vi "DUTResultsDialogSequential.vi"(5 "Left Coordinate":i16, 7 "Top Coordinate":i16, 8 "error in (no error)":errorcluster, 9 "MessageTxt":string, 11 "Value":string) -> (0 "error out":errorcluster)   [LabVIEW 2021]
doc: "Display DUT results banner for Pass, Fail, Error or Terminate."
panel:
  out "MssgText":string
  out "Message":string
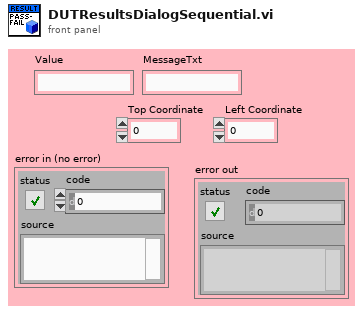
[diagram p1: front panel]
types:
  T1 = typedef "imagedata.ctl" = cluster{"image type":i32, "image depth":i32, "image":u8[], "mask":u8[], "colors":u32[], "Rectangle":cluster{"left":i16, "top":i16, "right":i16, "bottom":i16}}
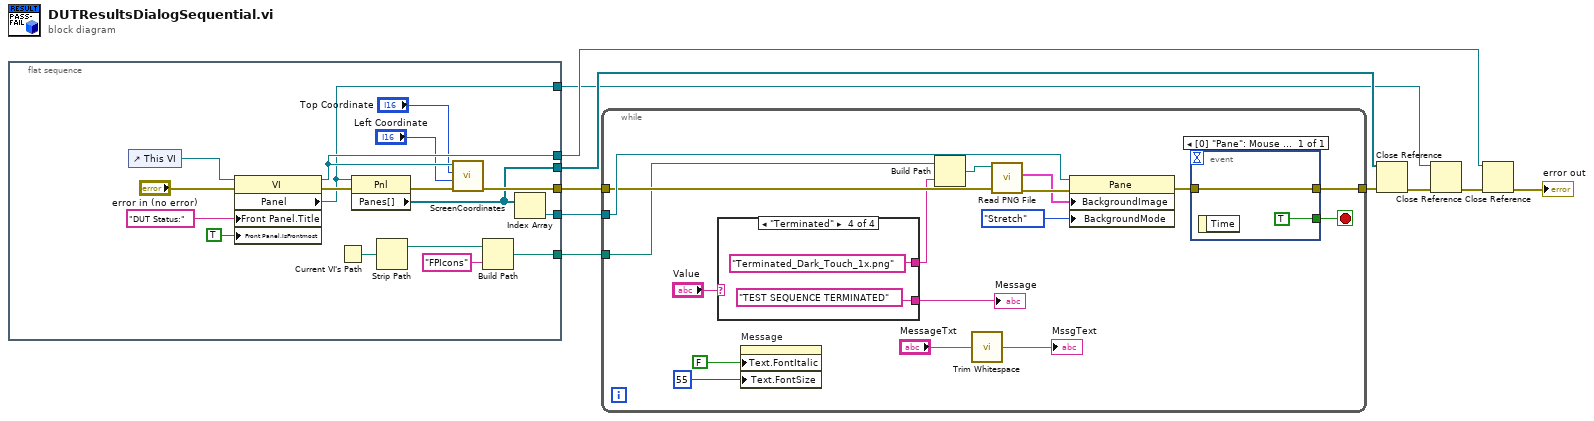
[diagram p0: block diagram]
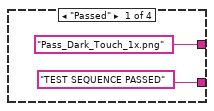
[diagram p2: hidden frame]
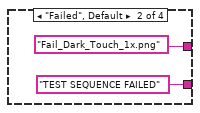
[diagram p3: hidden frame]
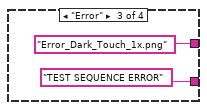
[diagram p4: hidden frame]
diagram:
  n1 = flat-sequence {
    tunnel: [w27] -> w8
    tunnel: [w24] -> w2
    tunnel: [w19] -> w7
    tunnel: [w16] -> w6
    tunnel: [w14] -> w5
    tunnel: [w13] -> w1
    frame #0 {
      n2 = control-ref of="This VI"() -> (w21:refnum<vi>)
      n3 = property class="VI"(reference=w21, error in="error in (no error)", "Front Panel.Title"="DUT Status:" ("Front Panel Window:Title"), "Front Panel.IsFrontmost"=TRUE ("Front Panel Window:Is Frontmost")) -> (reference out=w24:refnum<vi>, error out=w26:errorcluster, "Panel"=w13:refnum<vi>)
      n4 = Current VI's Path() -> (path=w18:path)
      n5 = property class="Pnl"(reference=w13, error in=w26) -> (error out=w20:errorcluster, "Panes[]"=w14:refnum<vi>[])  [unwired: 1 out]
      n6 = Strip Path(path=w18) -> (stripped path=w15:path)  [unwired: 1 out]
      n7 = call "ScreenCoordinates.vi"("error in (no error)"=w20, "Left Coordinate"="Left Coordinate", "Top Coordinate"="Top Coordinate", "ThisVI"=w24) -> ("error out"=w27:errorcluster)  [unwired: 6 in, 1 out]
      n8 = Build Path(base path=w15, name or relative path="FPIcons") -> (appended path=w16:path)
      n9 = Index Array(array=w14) -> (element=w19:refnum<vi>)  [unwired: 1 in]
    }
  }
  n10 = while {
    tunnel: [w31] -> w10
    tunnel: w8 -> [w39]
    tunnel: w7 -> [w41]
    tunnel: w6 -> [w35]
    stop <- w30 stop-if-true
    n11 = case shown="\"Terminated\"" "Value" {
      tunnel: ["TEST SEQUENCE PASSED" "TEST SEQUENCE FAILED" "TEST SEQUENCE ERROR" "TEST SEQUENCE TERMINATED"] -> w37
      tunnel: ["Pass_Dark_Touch_1x.png" "Fail_Dark_Touch_1x.png" "Error_Dark_Touch_1x.png" "Terminated_Dark_Touch_1x.png"] -> w34
      frame "Passed" {
      }
      frame "Failed", Default {
      }
      frame "Error" {
      }
      frame "Terminated" {
      }
    }
    "Message" <- w37
    n12 = property on="Message" class="Str"("Text.FontItalic"=FALSE ("Text.Font:Bold"), "Text.FontSize"=u32 55 ("Text.Font:Size")) -> ()  [unwired: 2 in, 2 out]
    n13 = Build Path(base path=w35, name or relative path=w34) -> (appended path=w33:path)
    n14 = call <vilib>:"Trim Whitespace.vi"("string"="MessageTxt") -> ("trimmed string"=→"MssgText":string)  [unwired: 1 in]
    n15 = call <vilib>:"Read PNG File.vi"("error in (no error)"=w39, "path to PNG file"=w33) -> ("error out"=w38:errorcluster, "image data"=w36:T1)  [unwired: 7 in, 1 out]
    n16 = property class="Pane"(reference=w41, error in=w38, "BackgroundImage"=w36, "BackgroundMode"=enum16{"Stretch", "Center", "Tile"}."Stretch" ("Background Mode")) -> (error out=w32:errorcluster)  [unwired: 1 out]
    n17 = event shown="[0] \"Pane\": Mouse Down" {
      selector: _ -> [_]
      dyn-events: _ -> [_]
      timeout: _ -> [_]
      tunnel: w32 -> [w46]
      tunnel: [w46] -> w31
      tunnel: [TRUE] -> w30
      event Mouse Down {
        n18 = event-data() -> ()  [unwired: 1 in, 1 out]
      }
    }
  }
  n19 = Close Reference(reference=w5, error in (no error)=w10) -> (error out=w9:errorcluster)
  n20 = Close Reference(reference=w1, error in (no error)=w9) -> (error out=w4:errorcluster)
  n21 = Close Reference(reference=w2, error in (no error)=w4) -> (error out=→"error out":errorcluster)
